vi "Read Count.vi"(8 "error in (no error)":errorcluster, 11 "Count Response Message in":refnum<class "Count Response Message.lvclass">) -> (0 "error out":errorcluster, 2 "Count":u32, 3 "Count Response Message out":refnum<class "Count Response Message.lvclass">)   [LabVIEW 2017, in "Count Response Message.lvclass"]
uses:
  Count Response Message.lvclass
  Count Response Message.lvclass/Count Response Message.ctl
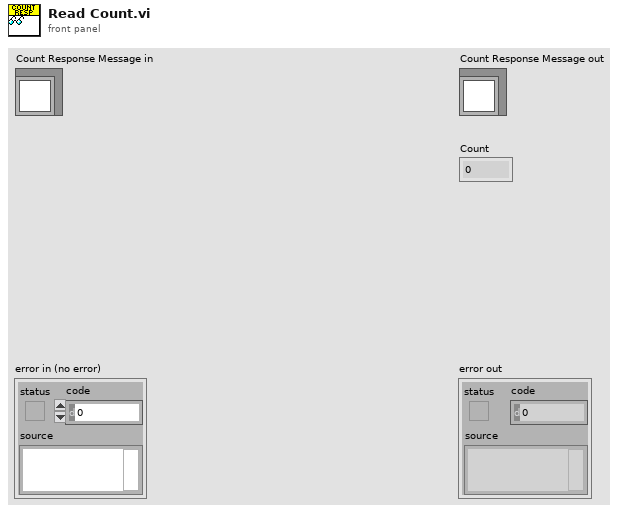
[diagram p1: front panel]
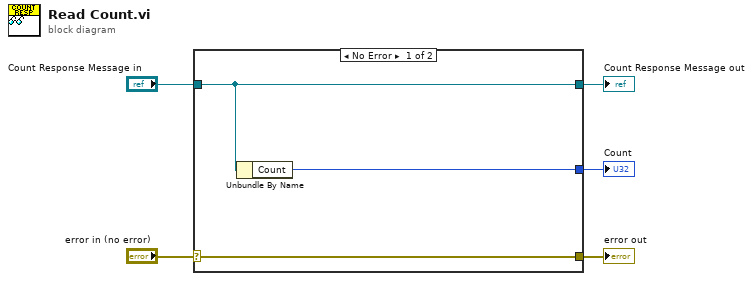
[diagram p0: block diagram]
diagram:
  n1 = case shown="No Error" "error in (no error)" {
    selector: "error in (no error)" -> [w8 w9]
    tunnel: [w8 w9] -> w4
    tunnel: [w7 w10] -> w2
    tunnel: "Count Response Message in" -> [w7 w10]
    tunnel: [w6 _] -> w1
    frame No Error {
      n2 = Unbundle By Name(w7) -> ("Count"=w6:u32)
    }
    frame Error {
    }
  }
  "error out" <- w4
  "Count Response Message out" <- w2
  "Count" <- w1
